vi "Autonomous Independent.vi"() -> ()   [LabVIEW 2016]
doc: "This VI is called when autonomous begins, and will automatically be terminated when autonomous ends. You can carry out timed or sensor driven robot movement independently without needing to return to the caller."
uses:
  <vilib>/Rock Robotics/WPI/Relay/WPI_RelayValue.ctl
  <vilib>/Rock Robotics/WPI/Camera/WPI_CameraImageSize.ctl
  <vilib>/Rock Robotics/WPI/Utilities/WPI_GetSetVariantRefNum.vi
  <vilib>/Rock Robotics/Network Tables/NT Read String.vi
  <vilib>/Rock Robotics/Network Tables/NT Write Numeric Array.vi
  <vilib>/Rock Robotics/Network Tables/NT Write String.vi
  <vilib>/addons/control/pid/pid.llb/PID (DBL).vi
  <vilib>/addons/control/pid/NI_PID_pid.lvlib
panel:
  out "Numeric":i32
  out "Image 4":T1(plugin-control)
  out "Boolean 2":bool=TRUE
  out "x > 0? 2":bool
  out "x 4":sgl
  out "x 3":sgl
  out "Number of Matches (Shape Matching 1) 2":i32
  out "Image 2":T1(plugin-control)
  out "Image":T1(plugin-control)
  out "Number of Matches (Shape Matching 1)":i32
  out "x 2":sgl
  out "x":sgl
  out "x > 0?":bool
  out "Boolean":bool=TRUE
  out "x >= y?":bool
  out "x < y?":bool
  # "Be sure to right-click and choose Data Operations>>Make Current Value default if you want to save the array values with the VI"
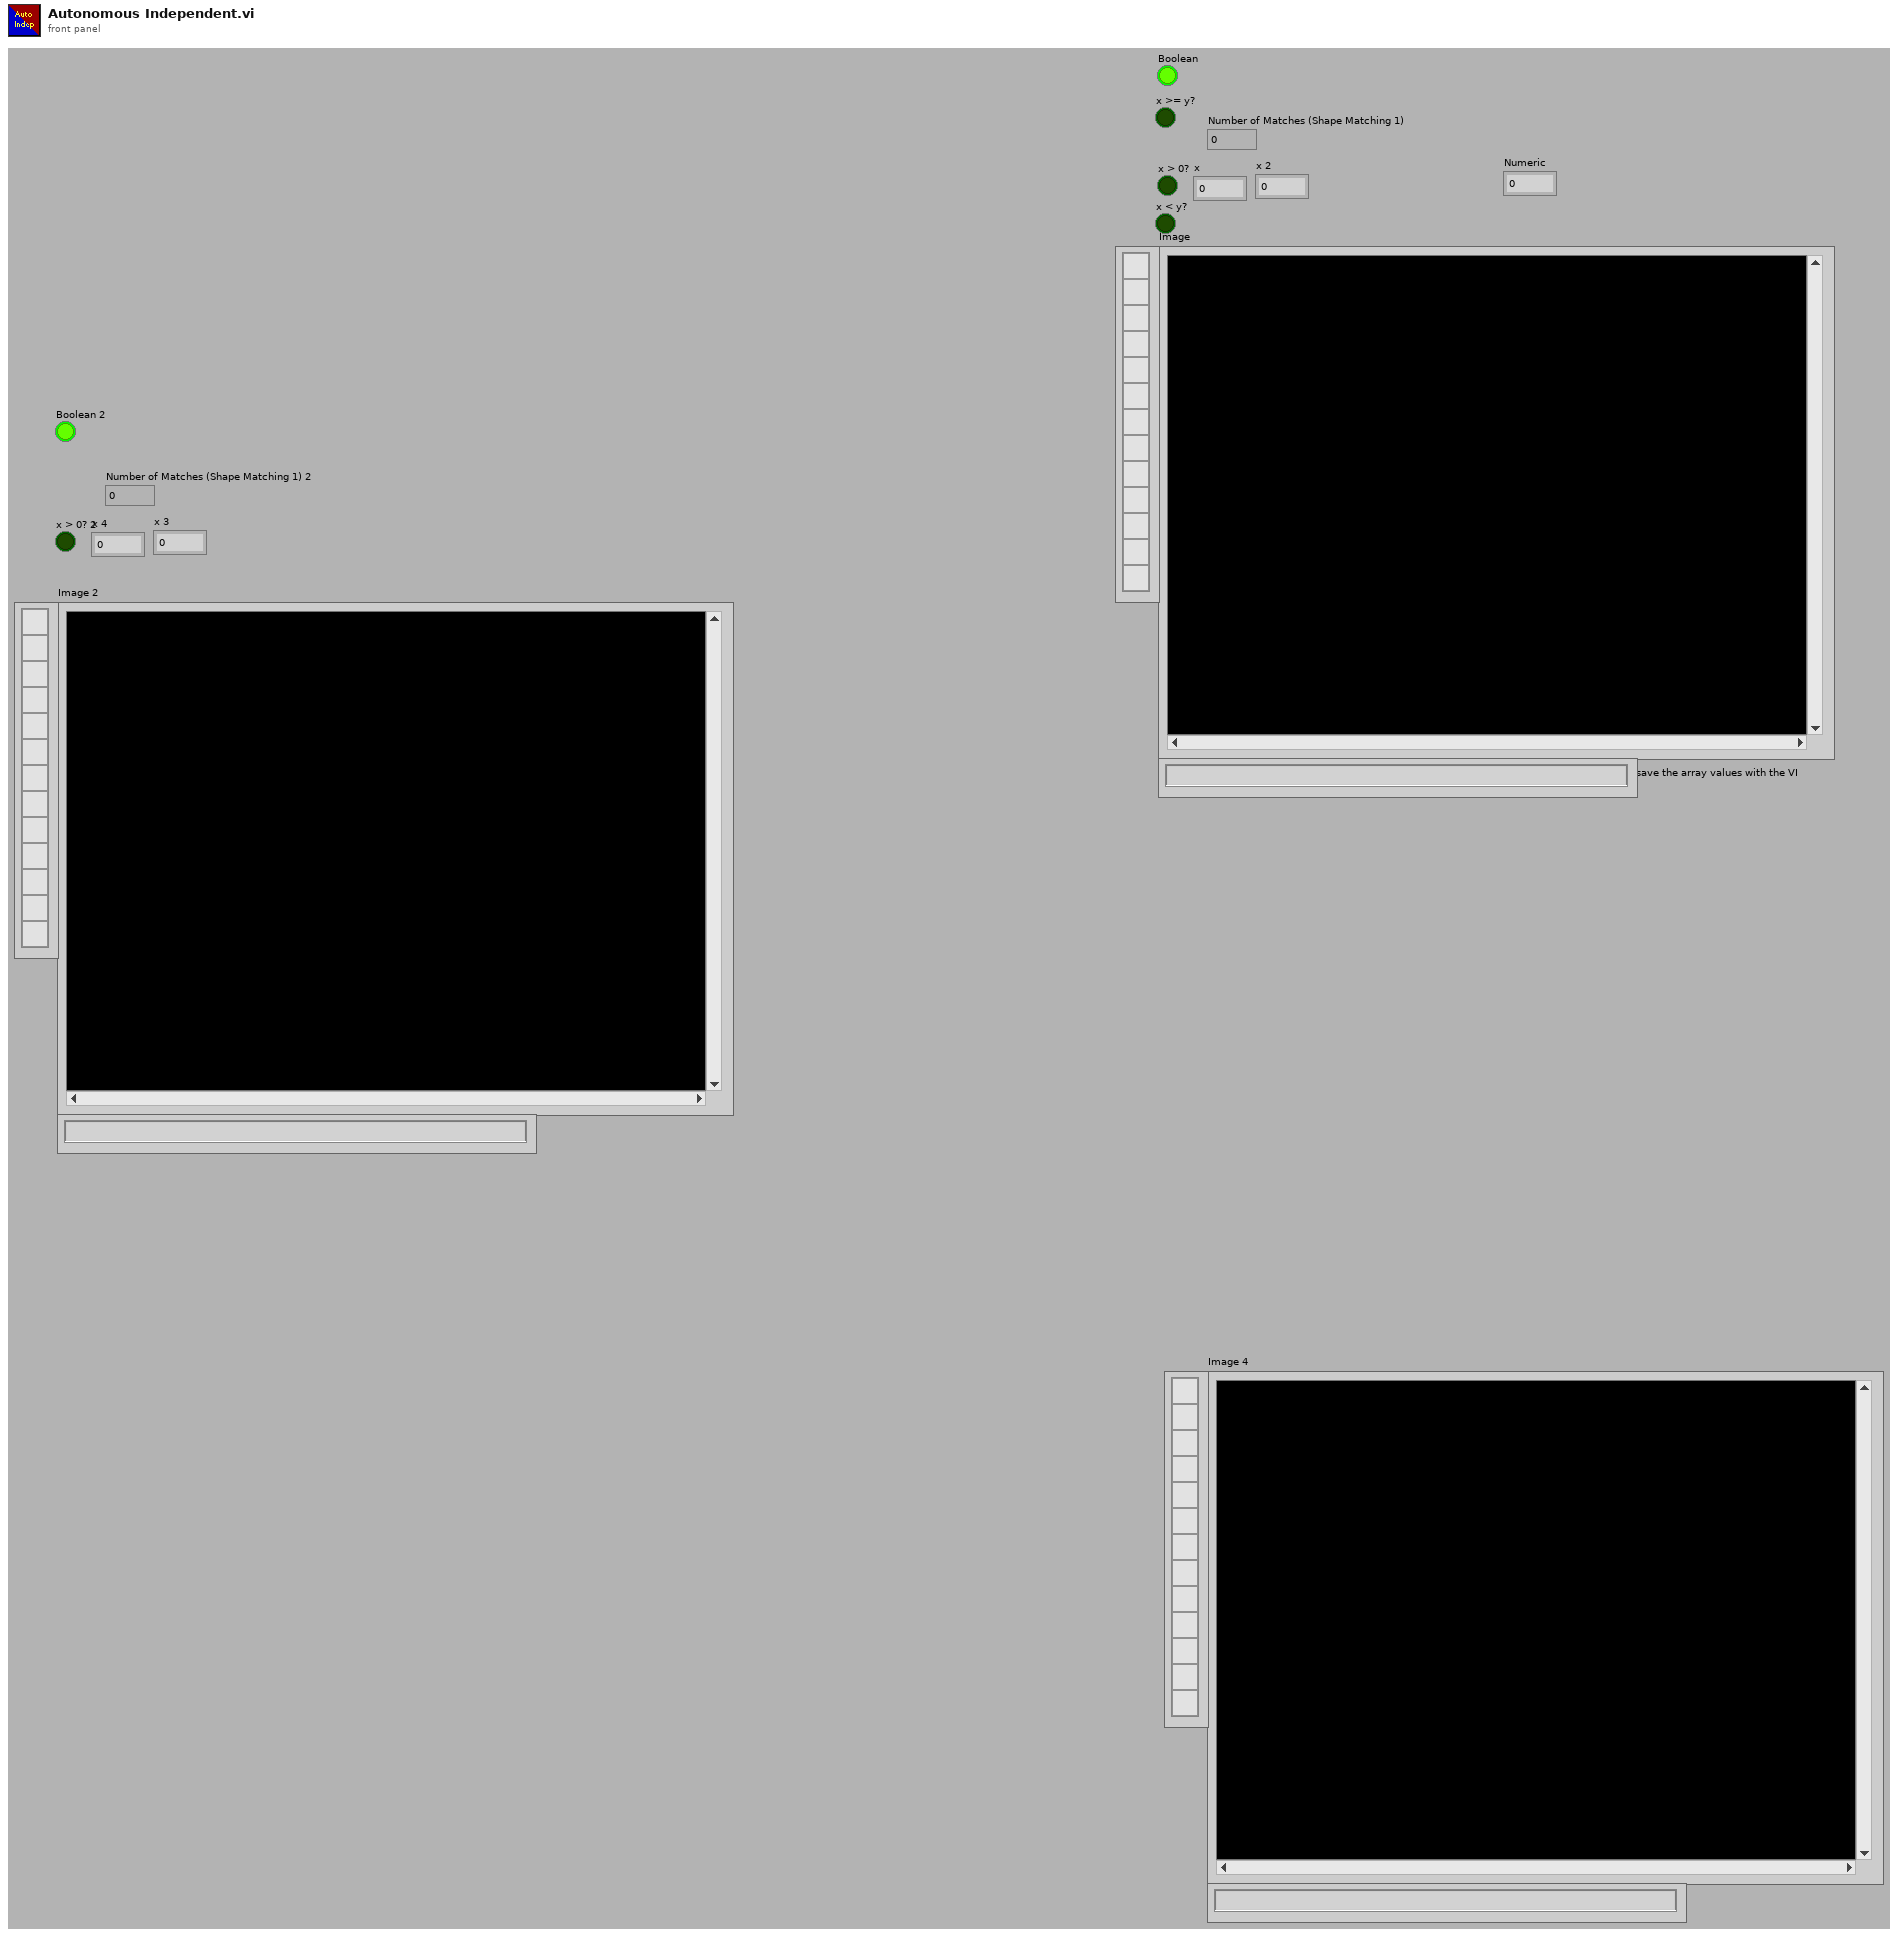
[diagram p1: front panel]
types:
  T1 = typedef "IMAQ Image.ctl" = refnum<image>
  T2 = typedef "WPI_DriverStationPositionInfo.ctl" = enum16{"1", "2", "3"}
  T3 = typedef "WPI_JoystickDevRef.ctl" = cluster{"Device":T4}
  T4 = typedef "WPI_JoystickDeviceEnum.ctl" = enum16{"USB 0", "USB 1", "USB 2", "USB 3", "USB 4", "USB 5"}
  T5 = typedef "WPI_RelayValue.ctl" = enum16{"Off", "On", "Forward", "Reverse"}
  T6 = cluster{"proportional gain (Kc)":dbl, "integral time (Ti, min)":dbl, "derivative time (Td, min)":dbl}
  T7 = typedef "WPI_CameraImageSize.ctl" = enum16{"640x480", "320x240", "160x120", "Custom"}
  T8 = typedef "WPI_EncoderDevRef.ctl" = cluster{"DevStatus":errorcluster, "EncoderIndex":T9, "CounterIndex":T10, "DistancePerCount":dbl, "Decoding Type":T11}
  T9 = typedef "FPGA_EncoderIdx.ctl" = enum8{"Enc 0", "Enc 1", "Enc 2", "Enc 3", "Enc 4", "Enc 5", "Enc 6", "Enc 7", "Invalid"}
  T10 = typedef "FPGA_CounterCtrSystemIndex.ctl" = enum8{"Ctr 0", "Ctr 1", "Ctr 2", "Ctr 3", "Ctr 4", "Ctr 5", "Ctr 6", "Ctr 7", "Invalid"}
  T11 = typedef "WPI_EncoderType.ctl" = enum16{"1x", "2x", "4x"}
  T12 = typedef "WPI_RelayDevRef.ctl" = cluster{"DevStatus":errorcluster, "Relay Channel":T13, "Relay Direction":T14}
  T13 = typedef "FPGA_DIORelayChannel.ctl" = enum8{"Relay 0", "Relay 1", "Relay 2", "Relay 3", "Invalid"}
  T14 = typedef "WPI_RelayDirection.ctl" = enum16{"Both directions", "Forward only", "Reverse only"}
  T15 = typedef "WPI_RobotDriveDevRef.ctl" = cluster{"DevStatus":errorcluster, "Motors[]":T16[], "Square Inputs":bool, "Max Output":dbl}
  T16 = typedef "WPI_MotorControlDeviceRef.ctl" = cluster{"DeviceStatus":errorcluster, "Type":T17, "PWM":cluster{"PWM Channel":T18, "DeadBand":T19}, "CAN":cluster{"Device Number":u8, "SetOutput VI Ref":variant, "GetOutput VI Ref":variant, "Enable VI Ref":variant, "Disable VI Ref":variant, "Data":variant}, "Invert":bool}
  T17 = typedef "WPI_MotorControlType.ctl" = enum16{"PWM", "CAN"}
  T18 = typedef "FPGA_DIOPWMChannel.ctl" = enum8{"PWM 0", "PWM 1", "PWM 2", "PWM 3", "PWM 4", "PWM 5", "PWM 6", "PWM 7", "PWM 8", "PWM 9", "PWM MXP 0", "PWM MXP 1", "PWM MXP 2", "PWM MXP 3", "PWM MXP 4", "PWM MXP 5", "PWM MXP 6", "PWM MXP 7", "PWM MXP 8", "PWM MXP 9", "Invalid"}
  T19 = typedef "WPI_PWMDeadband.ctl" = cluster{"Name":string, "maxPositivePwm":i32, "minPositivePwm":i32, "centerPwm":i32, "maxNegativePwm":i32, "minNegativePwm":i32, "angularRange":u16}
  T20 = typedef "WPI_GyroDevRef.ctl" = cluster{"DevStatus":errorcluster, "Analog Channel":T21, "Offset":dbl, "Gain (VoltsPerDegree/Second)":dbl, "Gyro Type":enum16{"Analog", "XRS450"}, "Handle":i32, "SPI Bus":T22, "Device Found":bool, "Sample Rate":dbl, "Calibrate On Open":bool}
  T21 = typedef "FPGA_AIChannel.ctl" = enum8{"AI 0", "AI 1", "AI 2", "AI 3", "AI MXP 0", "AI MXP 1", "AI MXP 2", "AI MXP 3", "Invalid"}
  T22 = typedef "spi_bus.ctl" = enum16{"SPI On-Board, CS0", "SPI On-Board, CS1", "SPI On-Board, CS2", "SPI On-Board, CS3", "SPI MXP", "Invalid"}
  T23 = typedef "Image Type" = u32
  T24 = typedef "WPI_CameraDevRef.ctl" = cluster{"Camera Address":string, "CameraStatus":errorcluster}
  T25 = cluster{"Global Rectangle":cluster{"x1Left":i32, "y1Top":i32, "x2Right":i32, "y2Bottom":i32}, "Centroid":cluster{"x":sgl, "y":sgl}, "Object Size":u32, "Score":dbl}[]
  T26 = cluster{"Global Rectangle":cluster{"x1Left":i32, "y1Top":i32, "x2Right":i32, "y2Bottom":i32}, "Centroid":cluster{"x":sgl, "y":sgl}, "Object Size":u32, "Score":dbl}
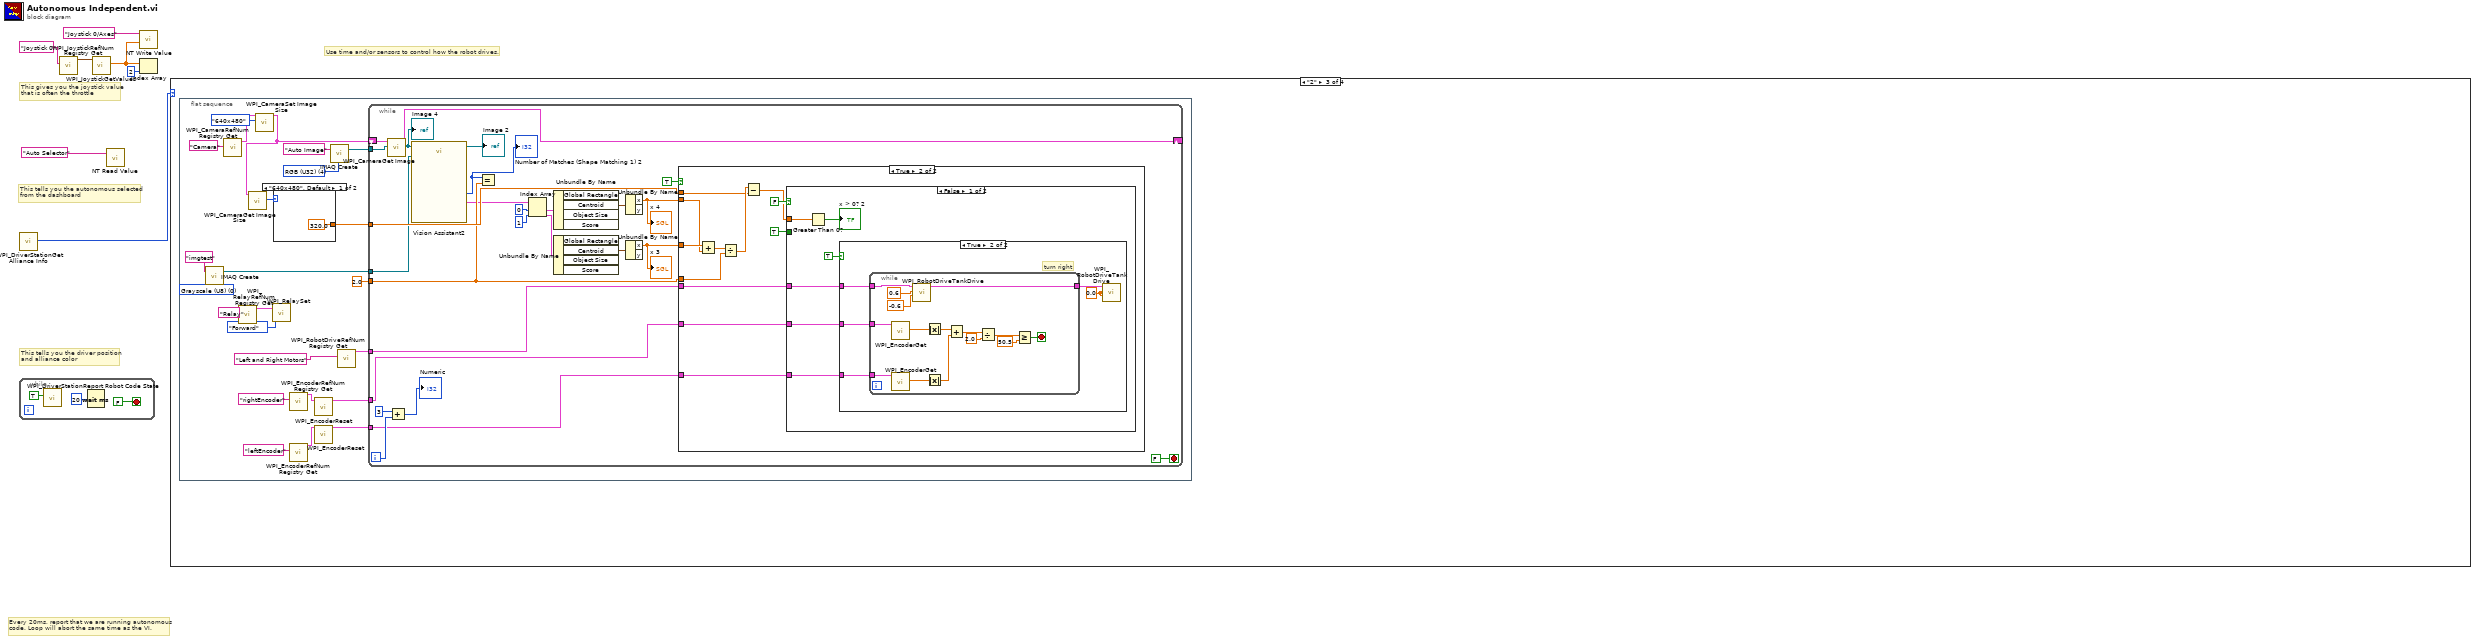
[diagram p0: block diagram]
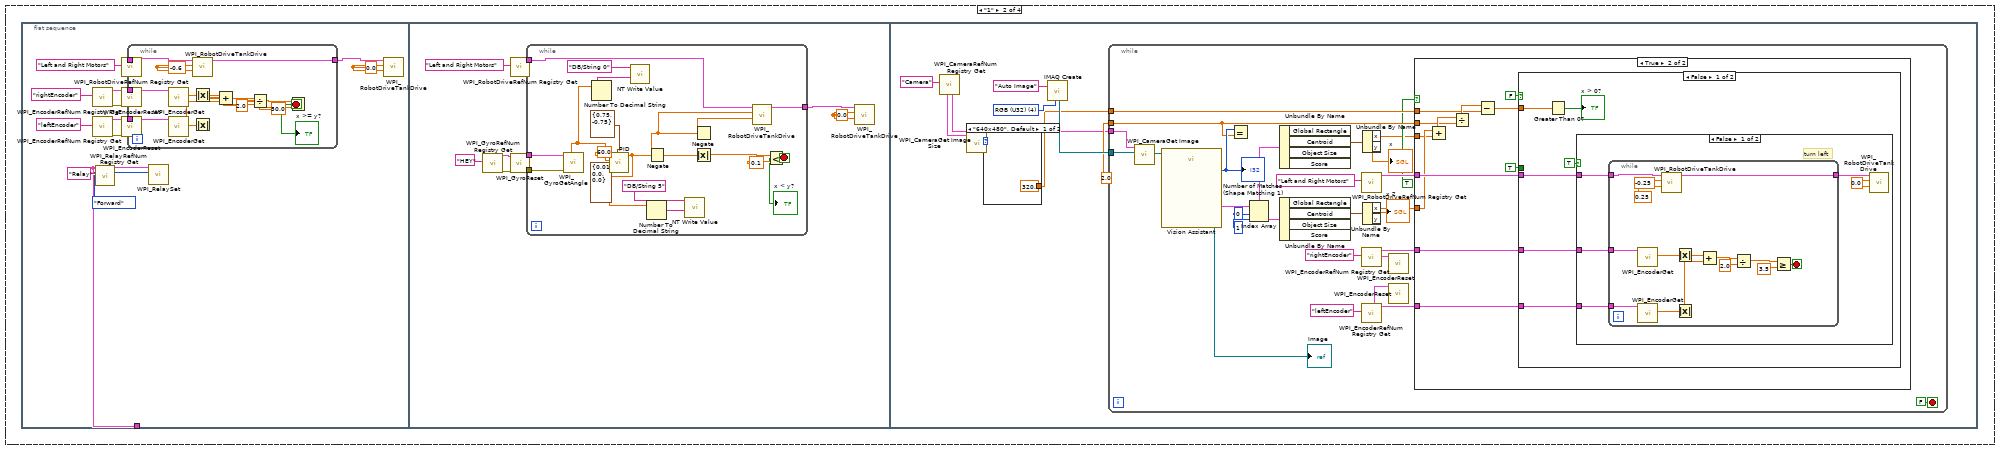
[diagram p3: hidden frame]
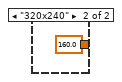
[diagram p4: hidden frame]
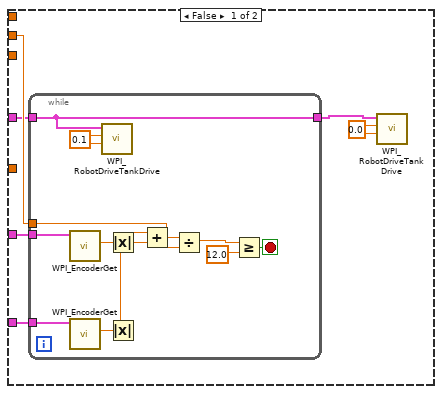
[diagram p5: hidden frame]
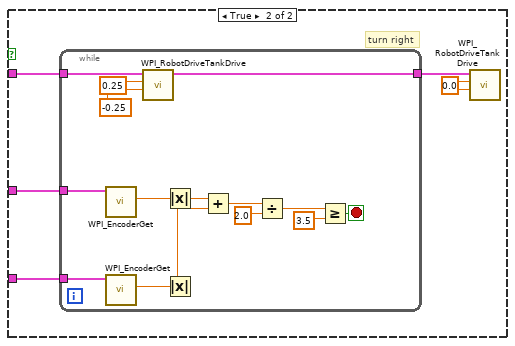
[diagram p6: hidden frame]
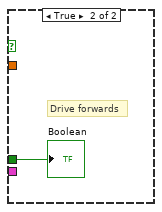
[diagram p7: hidden frame]
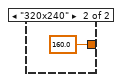
[diagram p8: hidden frame]
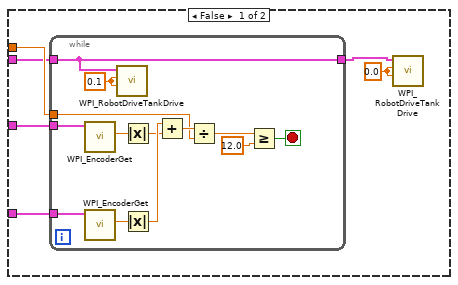
[diagram p9: hidden frame]
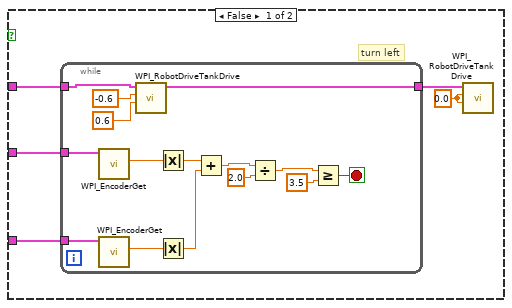
[diagram p10: hidden frame]
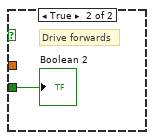
[diagram p11: hidden frame]
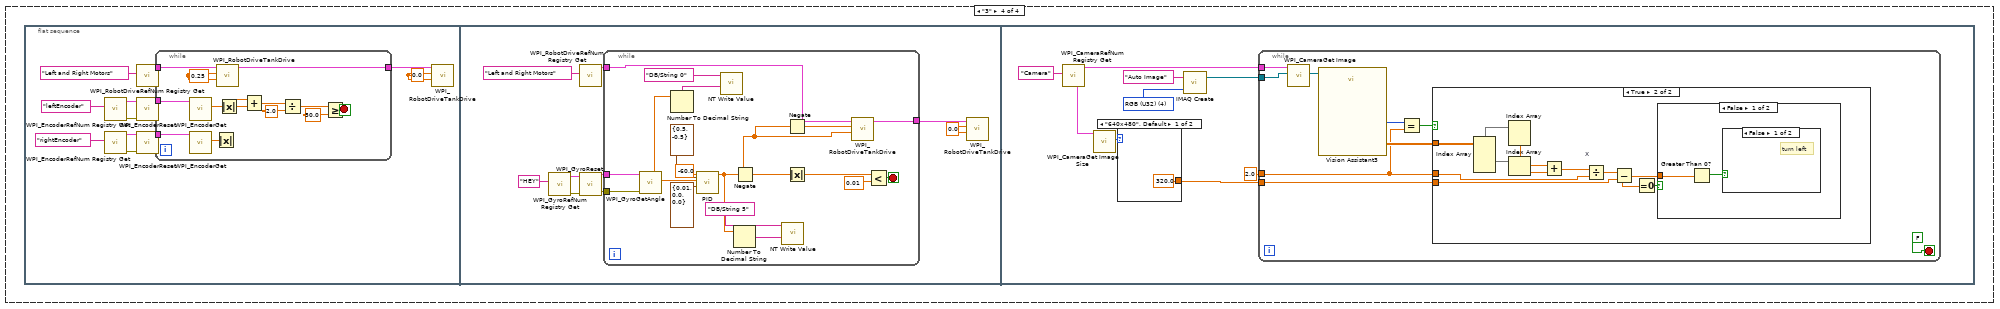
[diagram p12: hidden frame]
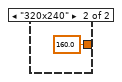
[diagram p13: hidden frame]
diagram:
  # "This tells you the autonomous selected\nfrom the dashboard"
  # "Every 20ms, report that we are running autonomous\ncode. Loop will abort the same time as the VI."
  # "This gives you the joystick value\nthat is often the throttle"
  # "Use time and/or sensors to control how the robot drives."
  # "This tells you the driver position\nand alliance color"
  n1 = while {
    stop <- FALSE stop-if-true
    n2 = call <vilib>:"WPI_DriverStationReport Robot Code State.vi"("Autonomous"=TRUE) -> ()  [unwired: 10 in, 1 out]
    n3 = Wait (ms)(milliseconds to wait=u32 20) -> ()  [unwired: 1 out]
  }
  n4 = call <vilib>:"WPI_DriverStationGet Alliance Info.vi"() -> ("Position"=w1:T2)  [unwired: 11 out]
  n5 = call <vilib>:"WPI_JoystickRefNum Registry Get.vi"("refnum name"="Joystick 0") -> ("JoystickDevRef"=w6:T3)  [unwired: 1 in, 9 out]
  n6 = call <vilib>:"WPI_JoystickGetValues.vi"("JoystickDevRef"=w6) -> ("Axes"=w3:dbl[])  [unwired: 6 in, 4 out]
  n7 = call-poly <vilib>:"NT Read Value.vi"("Name"="Auto Selector") -> ()  [unwired: 9 in, 2 out]
  n8 = call-poly <vilib>:"NT Write Value.vi"("Numeric Array"=w3, "Name"="Joystick 0/Axes") -> ()  [unwired: 9 in, 1 out]
  n9 = Index Array(array=w3, index=2) -> ()  [unwired: 1 out]
  n10 = case shown="\"2\"" w1 {
    frame Default {
      # "You can put your main auto here, or you can right-click on the case and make any\nother frame be the default case."
      # "This is the frame that will execute if no selection is made, or if it is not recognized"
    }
    frame "1" {
      n11 = flat-sequence {
        tunnel: [w11] -> _
        frame #0 {
          w14 = 0.0 ("Left axis value")
          n12 = call <vilib>:"WPI_EncoderRefNum Registry Get.vi"("refnum name"="rightEncoder") -> ("error out"=w20:errorcluster, "EncoderDevRef"=w21:T8)  [unwired: 9 in]
          n13 = call <vilib>:"WPI_EncoderRefNum Registry Get.vi"("refnum name"="leftEncoder") -> ("error out"=w23:errorcluster, "EncoderDevRef"=w22:T8)  [unwired: 9 in]
          n14 = call <vilib>:"WPI_RelayRefNum Registry Get.vi"("refnum name"="Relay") -> ("RelayDevRef"=w11:T12)  [unwired: 9 in, 1 out]
          n15 = call <vilib>:"WPI_RobotDriveRefNum Registry Get.vi"("refnum name"="Left and Right Motors") -> ("RobotDriveDevRef"=w16:T15)  [unwired: 9 in, 1 out]
          n16 = call <vilib>:"WPI_EncoderReset.vi"("error in (no error)"=w20, "EncoderDevRef"=w21) -> ("EncoderDevRef"=w19:T8)  [unwired: 8 in, 1 out]
          n17 = call <vilib>:"WPI_EncoderReset.vi"("error in (no error)"=w23, "EncoderDevRef"=w22) -> ("EncoderDevRef"=w18:T8)  [unwired: 8 in, 1 out]
          n18 = while {
            tunnel: w19 -> [w39]
            tunnel: w18 -> [w38]
            tunnel: w16 -> [w31]
            tunnel: [w29] -> w15
            stop <- w26 stop-if-true
            w30 = -0.6 ("Left axis value")
            n19 = call <vilib>:"WPI_EncoderGet.vi"("EncoderDevRef"=w39) -> ("Distance"=w37:dbl)  [unwired: 5 in, 5 out]
            n20 = call <vilib>:"WPI_EncoderGet.vi"("EncoderDevRef"=w38) -> ("Distance"=w36:dbl)  [unwired: 5 in, 5 out]
            n21 = call <vilib>:"WPI_RobotDriveTankDrive.vi"("Right axis value"=w30, "Left axis value"=w30, "RobotDriveDevRef"=w31) -> ("RobotDriveDevRef"=w29:T15)  [unwired: 6 in, 2 out]
            n22 = Absolute Value(x=w37) -> (abs(x)=w27:dbl)
            n23 = Absolute Value(x=w36) -> (abs(x)=w28:dbl)
            n24 = Add(x=w27, y=w28) -> (x+y=w35:dbl)
            n25 = Divide(x=w35, y=2.0) -> (x/y=w33:dbl)
            n26 = Greater Or Equal?(x=w33, y=50.0) -> (x >= y?=w26:bool)
            "x >= y?" <- w26
          }
          n27 = call <vilib>:"WPI_RelaySet.vi"("RelayValue"=WPI_RelayValue."Forward", "RelayDevRef"=w11) -> ()  [unwired: 8 in, 2 out]
          n28 = call <vilib>:"WPI_RobotDriveTankDrive.vi"("Right axis value"=w14, "Left axis value"=w14, "RobotDriveDevRef"=w15) -> ()  [unwired: 6 in, 3 out]
        }
        frame #1 {
          w41 = 0.0 ("Right axis value")
          n29 = call <vilib>:"WPI_GyroRefNum Registry Get.vi"("refnum name"="HEY") -> ("error out"=w47:errorcluster, "GyroDevRef"=w46:T20)  [unwired: 9 in]
          n30 = call <vilib>:"WPI_RobotDriveRefNum Registry Get.vi"("refnum name"="Left and Right Motors") -> ("RobotDriveDevRef"=w43:T15)  [unwired: 9 in, 1 out]
          n31 = call <vilib>:"WPI_GyroReset.vi"("error in"=w47, "GyroDevRef"=w46) -> ("error out"=w45:errorcluster, "GyroDevRef"=w44:T20)  [unwired: 8 in]
          n32 = while {
            tunnel: w45 -> [w66]
            tunnel: w44 -> [w65]
            tunnel: w43 -> [w61]
            tunnel: [w54] -> w42
            stop <- w58 stop-if-true
            n33 = call <vilib>:"WPI_GyroGetAngle.vi"("error in"=w66, "GyroDevRef"=w65) -> ("Angle"=w55:dbl)  [unwired: 5 in, 4 out]
            n34 = Number To Decimal String(number=w55) -> (decimal integer string=w57:string)  [unwired: 1 in]
            n35 = call-poly <vilib>:"PID.vi"("output range"=cluster{"output high":dbl, "output low":dbl} {"output high"=0.75, "output low"=-0.75}, "PID gains"=T6 {"proportional gain (Kc)"=0.01, "integral time (Ti, min)"=0.0, "derivative time (Td, min)"=0.0}, "process variable"=w55, "setpoint"=60.0) -> ("output"=w51:dbl)  [unwired: 6 in, 1 out]
            n36 = call-poly <vilib>:"NT Write Value.vi"("String"=w57, "Name"="DB/String 0") -> ()  [unwired: 9 in, 1 out]
            n37 = Number To Decimal String(number=w51) -> (decimal integer string=w53:string)  [unwired: 1 in]
            n38 = Negate(x=w51) -> (-x=w49:dbl)
            n39 = call-poly <vilib>:"NT Write Value.vi"("String"=w53, "Name"="DB/String 5") -> ()  [unwired: 9 in, 1 out]
            n40 = Negate(x=w49) -> (-x=w50:dbl)
            n41 = Absolute Value(x=w49) -> (abs(x)=w60:dbl)
            n42 = call <vilib>:"WPI_RobotDriveTankDrive.vi"("Right axis value"=w50, "Left axis value"=w49, "RobotDriveDevRef"=w61) -> ("RobotDriveDevRef"=w54:T15)  [unwired: 6 in, 2 out]
            n43 = Less?(x=w60, y=0.1) -> (x < y?=w58:bool)
            "x < y?" <- w58
          }
          n44 = call <vilib>:"WPI_RobotDriveTankDrive.vi"("Right axis value"=w41, "Left axis value"=w41, "RobotDriveDevRef"=w42) -> ()  [unwired: 6 in, 3 out]
        }
        frame #2 {
          w73 = T23 4 items=["Grayscale (U8)", "Grayscale (I16)", "Grayscale (SGL)", "Complex (CSG)", "RGB (U32)", "HSL (U32)", "RGB (U64)"] ("Image Type")
          n45 = call <vilib>:"WPI_CameraRefNum Registry Get.vi"("refnum name"="Camera") -> ("CameraDevRef"=w68:T24)  [unwired: 9 in, 1 out]
          n46 = call <vilib>:"WPI_CameraGet Image Size.vi"("CameraDevRef"=w68) -> ("Image Size"=w67:T7)  [unwired: 7 in, 3 out]
          n47 = case shown="\"640x480\", Default" w67 {
            tunnel: [320.0 160.0] -> w70
            frame "640x480", Default {
            }
            frame "320x240" {
            }
          }
          n48 = call "IMAQ Create"("Image Name"="Auto Image", "Image Type"=w73) -> ("New Image"=w71:T1)  [unwired: 2 in, 2 out]
          n49 = while {
            tunnel: w68 -> [w100]
            tunnel: w71 -> [w99]
            tunnel: 2.0 -> [w94]
            tunnel: w70 -> [w95]
            stop <- FALSE stop-if-true
            n50 = call <vilib>:"WPI_CameraGet Image.vi"("Image"=w99, "CameraDevRef"=w100) -> ("Image Out"=w98:T1)  [unwired: 7 in, 2 out]
            n51 = call "Vision Assistant"("Image In"=w98) -> ("Image Out"=→"Image":T1, "Number of Matches (Shape Matching 1)"=w96:i32, "Shape Report (Shape Matching 1)"=w83:T25)  [unwired: 22 in, 2 out]
            "Number of Matches (Shape Matching 1)" <- w96
            n52 = Equal?(x=w96, y=w94) -> ()  [unwired: 1 out]
            n53 = Index Array(array=w83, index #1=0 ("index"), index #2=1 ("index")) -> (element #1=w81:T26, element #2=w85:T26)
            n54 = Unbundle By Name(w81) -> ("Centroid"=w80:cluster{"x":sgl, "y":sgl})  [unwired: 3 out]
            n55 = Unbundle By Name(w85) -> ("Centroid"=w84:cluster{"x":sgl, "y":sgl})  [unwired: 3 out]
            n56 = call <vilib>:"WPI_RobotDriveRefNum Registry Get.vi"("refnum name"="Left and Right Motors") -> ("RobotDriveDevRef"=w92:T15)  [unwired: 9 in, 1 out]
            n57 = call <vilib>:"WPI_EncoderRefNum Registry Get.vi"("refnum name"="rightEncoder") -> ("EncoderDevRef"=w87:T8)  [unwired: 9 in, 1 out]
            n58 = call <vilib>:"WPI_EncoderRefNum Registry Get.vi"("refnum name"="leftEncoder") -> ("EncoderDevRef"=w88:T8)  [unwired: 9 in, 1 out]
            n59 = Unbundle By Name(w80) -> ("x"=w78:sgl)  [unwired: 1 out]
            "x" <- w78
            n60 = Unbundle By Name(w84) -> ("x"=w79:sgl)  [unwired: 1 out]
            "x 2" <- w79
            n61 = call <vilib>:"WPI_EncoderReset.vi"("EncoderDevRef"=w87) -> ()  [unwired: 9 in, 2 out]
            n62 = call <vilib>:"WPI_EncoderReset.vi"("EncoderDevRef"=w88) -> ()  [unwired: 9 in, 2 out]
            n63 = case shown="True" TRUE {
              tunnel: w95 -> [_ w121]
              tunnel: w94 -> [w106 w123]
              tunnel: w92 -> [w105 w131]
              tunnel: w88 -> [w104 w129]
              tunnel: w87 -> [w103 w130]
              tunnel: w79 -> [_ w126]
              tunnel: w78 -> [_ w125]
              frame False {
                w101 = 0.0
                n64 = while {
                  tunnel: w104 -> [w119]
                  tunnel: w103 -> [w118]
                  tunnel: w106 -> [w116]
                  tunnel: w105 -> [w107]
                  tunnel: [w107] -> w102
                  stop <- w115 stop-if-true
                  w113 = 0.1
                  n65 = call <vilib>:"WPI_EncoderGet.vi"("EncoderDevRef"=w118) -> ("Distance"=w109:dbl)  [unwired: 5 in, 5 out]
                  n66 = call <vilib>:"WPI_EncoderGet.vi"("EncoderDevRef"=w119) -> ("Distance"=w112:dbl)  [unwired: 5 in, 5 out]
                  n67 = call <vilib>:"WPI_RobotDriveTankDrive.vi"("Right axis value"=w113, "Left axis value"=w113, "RobotDriveDevRef"=w107) -> ()  [unwired: 6 in, 3 out]
                  n68 = Absolute Value(x=w109) -> (abs(x)=w110:dbl)
                  n69 = Absolute Value(x=w112) -> (abs(x)=w111:dbl)
                  n70 = Add(x=w111, y=w110) -> (x+y=w117:dbl)
                  n71 = Divide(x=w117, y=w116) -> (x/y=w108:dbl)
                  n72 = Greater Or Equal?(x=w108, y=12.0) -> (x >= y?=w115:bool)
                }
                n73 = call <vilib>:"WPI_RobotDriveTankDrive.vi"("Right axis value"=w101, "Left axis value"=w101, "RobotDriveDevRef"=w102) -> ()  [unwired: 6 in, 3 out]
              }
              frame True {
                n74 = Add(x=w126, y=w125) -> (x+y=w124:sgl)
                n75 = Divide(x=w124, y=w123) -> (x/y=w122:dbl)
                n76 = Subtract(x=w122, y=w121) -> (x-y=w120:dbl)
                n77 = case shown="False" FALSE {
                  tunnel: w120 -> [w137 _]
                  tunnel: w131 -> [w136 _]
                  tunnel: w130 -> [w135 _]
                  tunnel: w129 -> [w134 _]
                  tunnel: TRUE -> [_ w178]
                  frame False {
                    n78 = Greater Than 0?(x=w137) -> (x > 0?=→"x > 0?":bool)
                    n79 = case shown="False" TRUE {
                      tunnel: w136 -> [w142 w162]
                      tunnel: w135 -> [w141 w161]
                      tunnel: w134 -> [w140 w160]
                      frame False {
                        w138 = 0.0 ("Right axis value")
                        # "turn left"
                        n80 = while {
                          tunnel: w142 -> [w157]
                          tunnel: w141 -> [w145]
                          tunnel: w140 -> [w154]
                          tunnel: [w143] -> w139
                          stop <- w146 stop-if-true
                          n81 = call <vilib>:"WPI_EncoderGet.vi"("EncoderDevRef"=w145) -> ("Distance"=w144:dbl)  [unwired: 5 in, 5 out]
                          n82 = call <vilib>:"WPI_EncoderGet.vi"("EncoderDevRef"=w154) -> ("Distance"=w153:dbl)  [unwired: 5 in, 5 out]
                          n83 = call <vilib>:"WPI_RobotDriveTankDrive.vi"("Right axis value"=0.25, "Left axis value"=-0.25, "RobotDriveDevRef"=w157) -> ("RobotDriveDevRef"=w143:T15)  [unwired: 6 in, 2 out]
                          n84 = Absolute Value(x=w144) -> (abs(x)=w152:dbl)
                          n85 = Absolute Value(x=w153) -> (abs(x)=w151:dbl)
                          n86 = Add(x=w152, y=w151) -> (x+y=w150:dbl)
                          n87 = Divide(x=w150, y=2.0) -> (x/y=w148:dbl)
                          n88 = Greater Or Equal?(x=w148, y=3.5) -> (x >= y?=w146:bool)
                        }
                        n89 = call <vilib>:"WPI_RobotDriveTankDrive.vi"("Right axis value"=w138, "Left axis value"=w138, "RobotDriveDevRef"=w139) -> ()  [unwired: 6 in, 3 out]
                      }
                      frame True {
                        w158 = 0.0 ("Right axis value")
                        # "turn right"
                        n90 = while {
                          tunnel: w162 -> [w177]
                          tunnel: w161 -> [w165]
                          tunnel: w160 -> [w174]
                          tunnel: [w163] -> w159
                          stop <- w166 stop-if-true
                          n91 = call <vilib>:"WPI_EncoderGet.vi"("EncoderDevRef"=w165) -> ("Distance"=w164:dbl)  [unwired: 5 in, 5 out]
                          n92 = call <vilib>:"WPI_EncoderGet.vi"("EncoderDevRef"=w174) -> ("Distance"=w173:dbl)  [unwired: 5 in, 5 out]
                          n93 = call <vilib>:"WPI_RobotDriveTankDrive.vi"("Right axis value"=-0.25, "Left axis value"=0.25, "RobotDriveDevRef"=w177) -> ("RobotDriveDevRef"=w163:T15)  [unwired: 6 in, 2 out]
                          n94 = Absolute Value(x=w164) -> (abs(x)=w172:dbl)
                          n95 = Absolute Value(x=w173) -> (abs(x)=w171:dbl)
                          n96 = Add(x=w172, y=w171) -> (x+y=w170:dbl)
                          n97 = Divide(x=w170, y=2.0) -> (x/y=w168:dbl)
                          n98 = Greater Or Equal?(x=w168, y=3.5) -> (x >= y?=w166:bool)
                        }
                        n99 = call <vilib>:"WPI_RobotDriveTankDrive.vi"("Right axis value"=w158, "Left axis value"=w158, "RobotDriveDevRef"=w159) -> ()  [unwired: 6 in, 3 out]
                      }
                    }
                  }
                  frame True {
                    # "Drive forwards"
                    "Boolean" <- w178
                  }
                }
              }
            }
          }
        }
      }
    }
    frame "2" {
      n100 = flat-sequence {
        frame #0 {
          w190 = T23 0 items=["Grayscale (U8)", "Grayscale (I16)", "Grayscale (SGL)", "Complex (CSG)", "RGB (U32)", "HSL (U32)", "RGB (U64)", "Grayscale (U16)"] ("Image Type")
          w201 = T23 4 items=["Grayscale (U8)", "Grayscale (I16)", "Grayscale (SGL)", "Complex (CSG)", "RGB (U32)", "HSL (U32)", "RGB (U64)"] ("Image Type")
          n101 = call "IMAQ Create"("Image Name"="imgtest", "Image Type"=w190) -> ("New Image"=w194:T1)  [unwired: 3 in, 1 out]
          n102 = call <vilib>:"WPI_CameraRefNum Registry Get.vi"("refnum name"="Camera") -> ("CameraDevRef"=w189:T24)  [unwired: 9 in, 1 out]
          n103 = call <vilib>:"WPI_RelayRefNum Registry Get.vi"("refnum name"="Relay") -> ("RelayDevRef"=w192:T12)  [unwired: 9 in, 1 out]
          n104 = call <vilib>:"WPI_CameraSet Image Size.vi"("Image Size"=WPI_CameraImageSize."640x480", "CameraDevRef"=w189) -> ("CameraDevRef Out"=w187:T24)  [unwired: 8 in, 1 out]
          n105 = call <vilib>:"WPI_CameraGet Image Size.vi"("CameraDevRef"=w187) -> ("Image Size"=w196:T7)  [unwired: 7 in, 3 out]
          n106 = call <vilib>:"WPI_RelaySet.vi"("RelayValue"=WPI_RelayValue."Forward", "RelayDevRef"=w192) -> ()  [unwired: 8 in, 2 out]
          n107 = case shown="\"640x480\", Default" w196 {
            tunnel: [320.0 160.0] -> w198
            frame "640x480", Default {
            }
            frame "320x240" {
            }
          }
          n108 = call <vilib>:"WPI_EncoderRefNum Registry Get.vi"("refnum name"="rightEncoder") -> ("EncoderDevRef"=w184:T8)  [unwired: 9 in, 1 out]
          n109 = call <vilib>:"WPI_EncoderRefNum Registry Get.vi"("refnum name"="leftEncoder") -> ("EncoderDevRef"=w183:T8)  [unwired: 9 in, 1 out]
          n110 = call <vilib>:"WPI_EncoderReset.vi"("EncoderDevRef"=w184) -> ("EncoderDevRef"=w180:T8)  [unwired: 9 in, 1 out]
          n111 = call <vilib>:"WPI_EncoderReset.vi"("EncoderDevRef"=w183) -> ("EncoderDevRef"=w179:T8)  [unwired: 9 in, 1 out]
          n112 = call "IMAQ Create"("Image Name"="Auto Image", "Image Type"=w201) -> ("New Image"=w199:T1)  [unwired: 2 in, 2 out]
          n113 = call <vilib>:"WPI_RobotDriveRefNum Registry Get.vi"("refnum name"="Left and Right Motors") -> ("RobotDriveDevRef"=w185:T15)  [unwired: 9 in, 1 out]
          n114 = while {
            tunnel: w199 -> [w214]
            tunnel: 2.0 -> [w227]
            tunnel: w198 -> [w228]
            tunnel: w194 -> [w215]
            shift-right: [w212] -> _
            shift-left: w187 -> [w230]
            tunnel: w185 -> [w207]
            tunnel: w180 -> [w206]
            tunnel: w179 -> [w205]
            i -> [w210]
            stop <- FALSE stop-if-true
            n115 = call <vilib>:"WPI_CameraGet Image.vi"("Image"=w214, "CameraDevRef"=w230) -> ("Image Out"=w213:T1, "CameraDevRef Out"=w212:T24)  [unwired: 7 in, 1 out]
            "Image 4" <- w213
            n116 = Add(x=3, y=w210) -> (x+y=→"Numeric":i32)
            n117 = call "Vision Assistant2"("Image In"=w213, "Image Dst"=w215) -> ("Image Out"=→"Image 2":T1, "Number of Matches (Shape Matching 1)"=w229:i32, "Shape Report (Shape Matching 1)"=w222:T25)  [unwired: 21 in, 2 out]
            "Number of Matches (Shape Matching 1) 2" <- w229
            n118 = Equal?(x=w229, y=w227) -> ()  [unwired: 1 out]
            n119 = Index Array(array=w222, index #1=0 ("index"), index #2=1 ("index")) -> (element #1=w220:T26, element #2=w224:T26)
            n120 = Unbundle By Name(w220) -> ("Centroid"=w219:cluster{"x":sgl, "y":sgl})  [unwired: 3 out]
            n121 = Unbundle By Name(w224) -> ("Centroid"=w223:cluster{"x":sgl, "y":sgl})  [unwired: 3 out]
            n122 = Unbundle By Name(w219) -> ("x"=w217:sgl)  [unwired: 1 out]
            "x 4" <- w217
            n123 = Unbundle By Name(w223) -> ("x"=w218:sgl)  [unwired: 1 out]
            "x 3" <- w218
            n124 = case shown="True" TRUE {
              tunnel: w228 -> [_ w252]
              tunnel: w227 -> [w236 w254]
              tunnel: w207 -> [w235 w250]
              tunnel: w205 -> [w234 w260]
              tunnel: w206 -> [w233 w261]
              tunnel: w218 -> [_ w257]
              tunnel: w217 -> [_ w256]
              frame False {
                w231 = 0.0
                n125 = while {
                  tunnel: w234 -> [w249]
                  tunnel: w233 -> [w248]
                  tunnel: w236 -> [w246]
                  tunnel: w235 -> [w237]
                  tunnel: [w237] -> w232
                  stop <- w245 stop-if-true
                  w243 = 0.1
                  n126 = call <vilib>:"WPI_EncoderGet.vi"("EncoderDevRef"=w248) -> ("Distance"=w239:dbl)  [unwired: 5 in, 5 out]
                  n127 = call <vilib>:"WPI_EncoderGet.vi"("EncoderDevRef"=w249) -> ("Distance"=w242:dbl)  [unwired: 5 in, 5 out]
                  n128 = call <vilib>:"WPI_RobotDriveTankDrive.vi"("Right axis value"=w243, "Left axis value"=w243, "RobotDriveDevRef"=w237) -> ()  [unwired: 6 in, 3 out]
                  n129 = Absolute Value(x=w239) -> (abs(x)=w240:dbl)
                  n130 = Absolute Value(x=w242) -> (abs(x)=w241:dbl)
                  n131 = Add(x=w241, y=w240) -> (x+y=w247:dbl)
                  n132 = Divide(x=w247, y=w246) -> (x/y=w238:dbl)
                  n133 = Greater Or Equal?(x=w238, y=12.0) -> (x >= y?=w245:bool)
                }
                n134 = call <vilib>:"WPI_RobotDriveTankDrive.vi"("Right axis value"=w231, "Left axis value"=w231, "RobotDriveDevRef"=w232) -> ()  [unwired: 6 in, 3 out]
              }
              frame True {
                n135 = Add(x=w257, y=w256) -> (x+y=w255:sgl)
                n136 = Divide(x=w255, y=w254) -> (x/y=w253:dbl)
                n137 = Subtract(x=w253, y=w252) -> (x-y=w251:dbl)
                n138 = case shown="False" FALSE {
                  tunnel: w251 -> [w267 _]
                  tunnel: w261 -> [w266 _]
                  tunnel: w260 -> [w265 _]
                  tunnel: TRUE -> [_ w308]
                  tunnel: w250 -> [w262 _]
                  frame False {
                    n139 = Greater Than 0?(x=w267) -> (x > 0?=→"x > 0? 2":bool)
                    n140 = case shown="True" TRUE {
                      tunnel: w262 -> [w272 w292]
                      tunnel: w266 -> [w271 w291]
                      tunnel: w265 -> [w270 w290]
                      frame False {
                        w268 = 0.0 ("Right axis value")
                        # "turn left"
                        n141 = while {
                          tunnel: w272 -> [w287]
                          tunnel: w271 -> [w275]
                          tunnel: w270 -> [w284]
                          tunnel: [w273] -> w269
                          stop <- w276 stop-if-true
                          n142 = call <vilib>:"WPI_EncoderGet.vi"("EncoderDevRef"=w275) -> ("Distance"=w274:dbl)  [unwired: 5 in, 5 out]
                          n143 = call <vilib>:"WPI_EncoderGet.vi"("EncoderDevRef"=w284) -> ("Distance"=w283:dbl)  [unwired: 5 in, 5 out]
                          n144 = call <vilib>:"WPI_RobotDriveTankDrive.vi"("Right axis value"=0.6, "Left axis value"=-0.6, "RobotDriveDevRef"=w287) -> ("RobotDriveDevRef"=w273:T15)  [unwired: 6 in, 2 out]
                          n145 = Absolute Value(x=w274) -> (abs(x)=w282:dbl)
                          n146 = Absolute Value(x=w283) -> (abs(x)=w281:dbl)
                          n147 = Add(x=w282, y=w281) -> (x+y=w280:dbl)
                          n148 = Divide(x=w280, y=2.0) -> (x/y=w278:dbl)
                          n149 = Greater Or Equal?(x=w278, y=3.5) -> (x >= y?=w276:bool)
                        }
                        n150 = call <vilib>:"WPI_RobotDriveTankDrive.vi"("Right axis value"=w268, "Left axis value"=w268, "RobotDriveDevRef"=w269) -> ()  [unwired: 6 in, 3 out]
                      }
                      frame True {
                        w288 = 0.0 ("Right axis value")
                        # "turn right"
                        n151 = while {
                          tunnel: w292 -> [w293]
                          tunnel: w291 -> [w296]
                          tunnel: w290 -> [w305]
                          tunnel: [w294] -> w289
                          stop <- w297 stop-if-true
                          n152 = call <vilib>:"WPI_EncoderGet.vi"("EncoderDevRef"=w296) -> ("Distance"=w295:dbl)  [unwired: 5 in, 5 out]
                          n153 = call <vilib>:"WPI_EncoderGet.vi"("EncoderDevRef"=w305) -> ("Distance"=w304:dbl)  [unwired: 5 in, 5 out]
                          n154 = call <vilib>:"WPI_RobotDriveTankDrive.vi"("Right axis value"=-0.6, "Left axis value"=0.6, "RobotDriveDevRef"=w293) -> ("RobotDriveDevRef"=w294:T15)  [unwired: 6 in, 2 out]
                          n155 = Absolute Value(x=w295) -> (abs(x)=w303:dbl)
                          n156 = Absolute Value(x=w304) -> (abs(x)=w302:dbl)
                          n157 = Add(x=w303, y=w302) -> (x+y=w301:dbl)
                          n158 = Divide(x=w301, y=2.0) -> (x/y=w299:dbl)
                          n159 = Greater Or Equal?(x=w299, y=50.5) -> (x >= y?=w297:bool)
                        }
                        n160 = call <vilib>:"WPI_RobotDriveTankDrive.vi"("Right axis value"=w288, "Left axis value"=w288, "RobotDriveDevRef"=w289) -> ()  [unwired: 6 in, 3 out]
                      }
                    }
                  }
                  frame True {
                    # "Drive forwards"
                    "Boolean 2" <- w308
                  }
                }
              }
            }
          }
        }
      }
    }
    frame "3" {
      n161 = flat-sequence {
        frame #0 {
          w310 = 0.0 ("Left axis value")
          n162 = call <vilib>:"WPI_EncoderRefNum Registry Get.vi"("refnum name"="leftEncoder") -> ("error out"=w318:errorcluster, "EncoderDevRef"=w317:T8)  [unwired: 9 in]
          n163 = call <vilib>:"WPI_EncoderRefNum Registry Get.vi"("refnum name"="rightEncoder") -> ("error out"=w315:errorcluster, "EncoderDevRef"=w316:T8)  [unwired: 9 in]
          n164 = call <vilib>:"WPI_RobotDriveRefNum Registry Get.vi"("refnum name"="Left and Right Motors") -> ("RobotDriveDevRef"=w311:T15)  [unwired: 9 in, 1 out]
          n165 = call <vilib>:"WPI_EncoderReset.vi"("error in (no error)"=w318, "EncoderDevRef"=w317) -> ("EncoderDevRef"=w313:T8)  [unwired: 8 in, 1 out]
          n166 = call <vilib>:"WPI_EncoderReset.vi"("error in (no error)"=w315, "EncoderDevRef"=w316) -> ("EncoderDevRef"=w314:T8)  [unwired: 8 in, 1 out]
          n167 = while {
            tunnel: w314 -> [w333]
            tunnel: w313 -> [w332]
            tunnel: w311 -> [w325]
            tunnel: [w323] -> w309
            stop <- w322 stop-if-true
            w324 = 0.25 ("Left axis value")
            n168 = call <vilib>:"WPI_EncoderGet.vi"("EncoderDevRef"=w332) -> ("Distance"=w330:dbl)  [unwired: 5 in, 5 out]
            n169 = call <vilib>:"WPI_EncoderGet.vi"("EncoderDevRef"=w333) -> ("Distance"=w331:dbl)  [unwired: 5 in, 5 out]
            n170 = Absolute Value(x=w331) -> ()  [unwired: 1 out]
            n171 = call <vilib>:"WPI_RobotDriveTankDrive.vi"("Right axis value"=w324, "Left axis value"=w324, "RobotDriveDevRef"=w325) -> ("RobotDriveDevRef"=w323:T15)  [unwired: 6 in, 2 out]
            n172 = Absolute Value(x=w330) -> (abs(x)=w321:dbl)
            n173 = Add(x=w321, y=w321) -> (x+y=w329:dbl)
            n174 = Divide(x=w329, y=2.0) -> (x/y=w327:dbl)
            n175 = Greater Or Equal?(x=w327, y=50.0) -> (x >= y?=w322:bool)
          }
          n176 = call <vilib>:"WPI_RobotDriveTankDrive.vi"("Right axis value"=w310, "Left axis value"=w310, "RobotDriveDevRef"=w309) -> ()  [unwired: 6 in, 3 out]
        }
        frame #1 {
          w335 = 0.0 ("Right axis value")
          n177 = call <vilib>:"WPI_GyroRefNum Registry Get.vi"("refnum name"="HEY") -> ("error out"=w341:errorcluster, "GyroDevRef"=w340:T20)  [unwired: 9 in]
          n178 = call <vilib>:"WPI_RobotDriveRefNum Registry Get.vi"("refnum name"="Left and Right Motors") -> ("RobotDriveDevRef"=w337:T15)  [unwired: 9 in, 1 out]
          n179 = call <vilib>:"WPI_GyroReset.vi"("error in"=w341, "GyroDevRef"=w340) -> ("error out"=w339:errorcluster, "GyroDevRef"=w338:T20)  [unwired: 8 in]
          n180 = while {
            tunnel: w339 -> [w360]
            tunnel: w338 -> [w359]
            tunnel: w337 -> [w355]
            tunnel: [w348] -> w336
            stop <- w352 stop-if-true
            n181 = call <vilib>:"WPI_GyroGetAngle.vi"("error in"=w360, "GyroDevRef"=w359) -> ("Angle"=w349:dbl)  [unwired: 5 in, 4 out]
            n182 = Number To Decimal String(number=w349) -> (decimal integer string=w351:string)  [unwired: 1 in]
            n183 = call-poly <vilib>:"PID.vi"("output range"=cluster{"output high":dbl, "output low":dbl} {"output high"=0.5, "output low"=-0.5}, "PID gains"=T6 {"proportional gain (Kc)"=0.01, "integral time (Ti, min)"=0.0, "derivative time (Td, min)"=0.0}, "process variable"=w349, "setpoint"=-60.0) -> ("output"=w345:dbl)  [unwired: 6 in, 1 out]
            n184 = call-poly <vilib>:"NT Write Value.vi"("String"=w351, "Name"="DB/String 0") -> ()  [unwired: 9 in, 1 out]
            n185 = Number To Decimal String(number=w345) -> (decimal integer string=w347:string)  [unwired: 1 in]
            n186 = Negate(x=w345) -> (-x=w343:dbl)
            n187 = call-poly <vilib>:"NT Write Value.vi"("String"=w347, "Name"="DB/String 5") -> ()  [unwired: 9 in, 1 out]
            n188 = Negate(x=w343) -> (-x=w344:dbl)
            n189 = Absolute Value(x=w343) -> (abs(x)=w354:dbl)
            n190 = call <vilib>:"WPI_RobotDriveTankDrive.vi"("Right axis value"=w343, "Left axis value"=w344, "RobotDriveDevRef"=w355) -> ("RobotDriveDevRef"=w348:T15)  [unwired: 6 in, 2 out]
            n191 = Less?(x=w354, y=0.01) -> (x < y?=w352:bool)
          }
          n192 = call <vilib>:"WPI_RobotDriveTankDrive.vi"("Right axis value"=w335, "Left axis value"=w335, "RobotDriveDevRef"=w336) -> ()  [unwired: 6 in, 3 out]
        }
        frame #2 {
          w367 = T23 4 items=["Grayscale (U8)", "Grayscale (I16)", "Grayscale (SGL)", "Complex (CSG)", "RGB (U32)", "HSL (U32)", "RGB (U64)"] ("Image Type")
          n193 = call <vilib>:"WPI_CameraRefNum Registry Get.vi"("refnum name"="Camera") -> ("CameraDevRef"=w362:T24)  [unwired: 9 in, 1 out]
          n194 = call <vilib>:"WPI_CameraGet Image Size.vi"("CameraDevRef"=w362) -> ("Image Size"=w361:T7)  [unwired: 7 in, 3 out]
          n195 = case shown="\"640x480\", Default" w361 {
            tunnel: [320.0 160.0] -> w364
            frame "640x480", Default {
            }
            frame "320x240" {
            }
          }
          n196 = call "IMAQ Create"("Image Name"="Auto Image", "Image Type"=w367) -> ("New Image"=w365:T1)  [unwired: 2 in, 2 out]
          n197 = while {
            tunnel: w362 -> [w379]
            tunnel: w365 -> [w378]
            tunnel: 2.0 -> [w371]
            tunnel: w364 -> [w372]
            stop <- FALSE stop-if-true
            n198 = call <vilib>:"WPI_CameraGet Image.vi"("Image"=w378, "CameraDevRef"=w379) -> ("Image Out"=w377:T1)  [unwired: 7 in, 2 out]
            n199 = call "Vision Assistant3"("Image In"=w377) -> ("Number of Particles (Particle Analysis 1)"=w375:i32, "Particle Measurements (Pixels) (Particle Analysis 1)"=w373:dbl[][])  [unwired: 22 in, 3 out]
            n200 = Equal?(x=w375, y=w371) -> (x = y?=w374:bool)
            n201 = case shown="True" w374 {
              tunnel: w373 -> [_ w383]
              tunnel: w372 -> [_ w382]
              tunnel: w371 -> [_ w381]
              frame False {
              }
              frame True {
                n202 = Index Array(array=w383) -> (element #1=w384:dbl[], element #2=w385:dbl[])  [unwired: 4 in]
                n203 = Index Array(array=w384) -> (element #1=w386:dbl)  [unwired: 2 in, 1 out]
                n204 = Index Array(array=w385) -> (element=w387:dbl)  [unwired: 1 in]
                n205 = Add(x=w386, y=w387) -> (x+y=w388:dbl)
                n206 = Divide "X"(x=w388, y=w381) -> (x/y=w389:dbl)
                n207 = Subtract(x=w389, y=w382) -> (x-y=w380:dbl)
                n208 = Equal To 0?(x=w380) -> (x = 0?=w390:bool)
                n209 = case shown="False" w390 {
                  tunnel: w380 -> [w392 _]
                  frame False {
                    n210 = Greater Than 0?(x=w392) -> (x > 0?=w391:bool)
                    n211 = case shown="False" w391 {
                      frame False {
                        # "turn left"
                      }
                      frame True {
                        # "turn right"
                      }
                    }
                  }
                  frame True {
                    # "Drive forwards"
                  }
                }
              }
            }
          }
        }
      }
    }
  }
